vi "Config Dev Stream.vi"(8 "error in":errorcluster, 10 "Stream (Normal)":i32(ring) items=["Normal", "Error"], 11 "VISA resource name":refnum<visa-resource-name>) -> (0 "error out":errorcluster, 3 "VISA resource name out":refnum<visa-resource-name>)   [LabVIEW 2019, in "Andeen-Hagerling 2700(400 firmware).lvlib"]
doc: "Selects which of the N or E streams is sent to the display and to remote systems after execution of a SINGLE, CONTINUOUS or FETCH command."
uses:
  Andeen-Hagerling 2700(400 firmware).lvlib
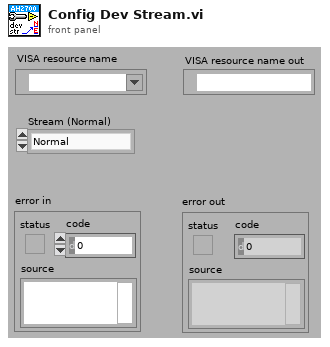
[diagram p1: front panel]
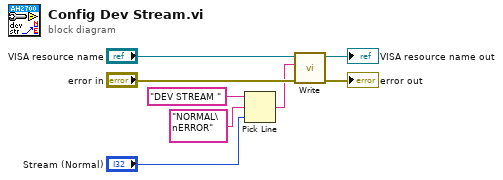
[diagram p0: block diagram]
diagram:
  n1 = Pick Line(string ("")="DEV STREAM " ("format string"), multi-line string="NORMAL\nERROR", line index="Stream (Normal)") -> (output string=w3:string)
  n2 = call "Write.vi"("error in"="error in", "command"=w3, "VISA resource name"="VISA resource name") -> ("error out"=→"error out":errorcluster, "VISA resource name out"=→"VISA resource name out":refnum<visa-resource-name>)  [unwired: 7 in]
